vi "Contour - Contour to Array Points.vi"(0 "Contour":T1) -> (4 "Array Points":i16[][](array[numeric]))   [LabVIEW 2014]
doc: "Conversion from Contour to Array Points"
uses:
  MSC Image_class/controls/Contour.ctl
  MSC Image_class/MSC Image.lvclass
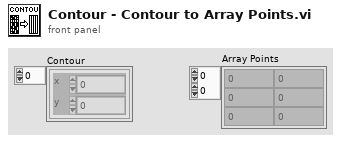
[diagram p1: front panel]
types:
  T1 = typedef "MSC Image.lvclass/Contour.ctl" = cluster{"x":i16, "y":i16}[]
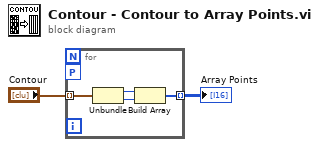
[diagram p0: block diagram]
diagram:
  n1 = for {
    tunnel: "Contour" -> [w6] mode=indexing
    tunnel: [w3] -> w2 mode=indexing
    workers-P: _ -> [_]
    n2 = Unbundle(w6) -> ("x"=w5:i16, "y"=w4:i16)
    n3 = Build Array(w5, w4) -> (w3:i16[])
  }
  "Array Points" <- w2
